vi "Execute.vi"(8 "error in (no error)":errorcluster, 9 "System in":refnum<class "System.lvclass">, 10 "Command in":refnum<class "Command.lvclass">, 11 "Shifter-HighSpeed in":refnum<class "Shifter-HighSpeed.lvclass">) -> (0 "error out":errorcluster, 2 "Next State":refnum<class "State.lvclass">, 3 "Shifter-HighSpeed out":refnum<class "Shifter-HighSpeed.lvclass">)   [LabVIEW 2013, in "Shifter-HighSpeed.lvclass"]
uses:
  Shifter-HighSpeed.lvclass
  Commands/Command/Command.lvclass
  Systems/System/System.lvclass
  State/State.lvclass
  Systems/Shifter/Shifter.lvclass
  Robot Global Data.vi
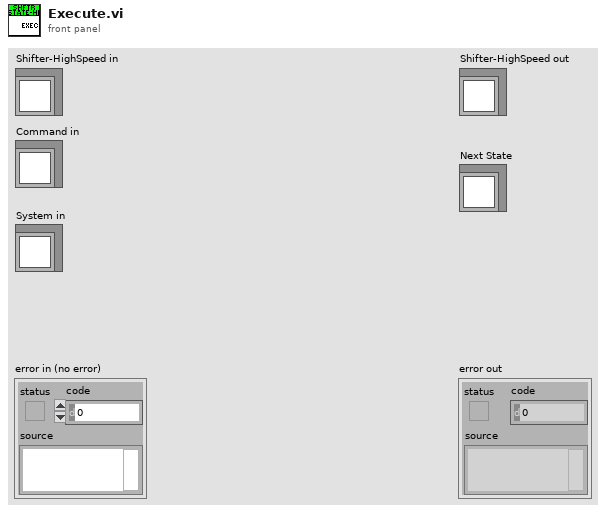
[diagram p1: front panel]
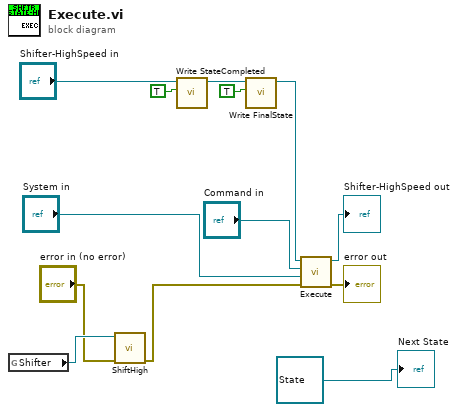
[diagram p0: block diagram]
diagram:
  n1 = global read "Robot Global Data.vi" "Shifter"() -> (w3:refnum<class "Shifter.lvclass">)
  n2 = call-dynamic "ShiftHigh.vi"("error in (no error)"="error in (no error)", "Shifter in"=w3) -> ("error out"=w1:errorcluster)  [unwired: 8 in, 1 out]
  n3 = call-dynamic "Write StateCompleted.vi"("StateCompleted"=TRUE, "State in"="Shifter-HighSpeed in") -> ("State out"=w10:refnum<class "Shifter-HighSpeed.lvclass">)  [unwired: 8 in, 1 out]
  n4 = call-dynamic "Write FinalState.vi"("FinalState"=TRUE, "State in"=w10) -> ("State out"=w8:refnum<class "Shifter-HighSpeed.lvclass">)  [unwired: 8 in, 1 out]
  n5 = call-parent "Execute.vi"("error in (no error)"=w1, "System in"="System in", "Command in"="Command in", "State in"=w8) -> ("error out"=→"error out":errorcluster, "State out"=→"Shifter-HighSpeed out":refnum<class "Shifter-HighSpeed.lvclass">)  [unwired: 5 in, 1 out]
  "Next State" <- refnum<class "State.lvclass"> refnum ("State.lvclass")
